vi "DL-Restore Configuration.vi"(11 "Error In":errorcluster) -> (8 "Config":T1={"Folder"=path "C:/Data", "Filestem"="Untitled", "Device"="", "Fs (Hz)"=50000.0, "T (s)"=120.0, "AI"=[], "frame size (s)"=1.0, ".wav file"=FALSE, "Trigger"=enum."Internal"}, 15 "error out":errorcluster)   [LabVIEW 2020]
uses:
  Typedefs/DL-Configuration.ctl
  Typedefs/DL-Channel Spec.ctl
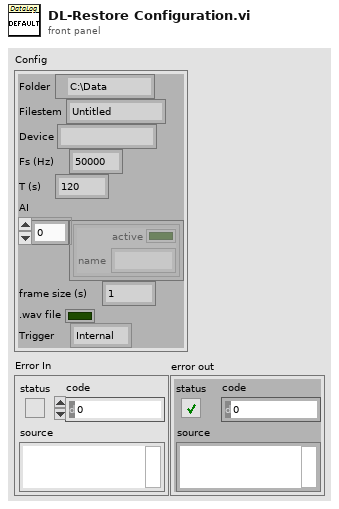
[diagram p1: front panel]
types:
  T1 = typedef "DL-Configuration.ctl" = cluster{"Folder":path, "Filestem":string, "Device":string, "Fs (Hz)":dbl, "T (s)":dbl, "AI":T2[], "frame size (s)":dbl, ".wav file":bool, "Trigger":enum16{"Internal", "External"}}
  T2 = typedef "DL-Channel Spec.ctl" = cluster{"active":bool, "name":string}
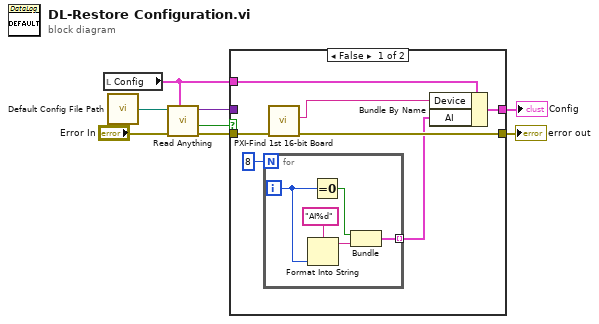
[diagram p0: block diagram]
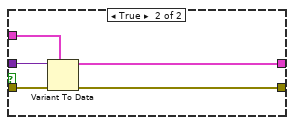
[diagram p2: hidden frame]
diagram:
  n1 = local read "Config"() -> (w3:T1)
  n2 = call "Default Config File Path.vi"() -> ("Default config file name"=w8:path)
  n3 = call "Read Anything.vi"("Type of Anything"=w3, "Error In"="Error In", "Path (dialog)"=w8) -> ("Error Out"=w4:errorcluster, "Found?"=w5:bool, "Anything"=w6:variant)  [unwired: 6 in]
  n4 = case shown="False" w5 {
    tunnel: w6 -> [_ w24]
    tunnel: w4 -> [w15 w25]
    tunnel: w3 -> [w14 w23]
    tunnel: [w12 w22] -> w2
    tunnel: [w11 w21] -> w1
    frame False {
      n5 = for {
        N: 8 -> [_]
        tunnel: [w16] -> w9 mode=indexing
        i -> [w18]
        n6 = Format Into String(format string="AI%d", w18) -> (resulting string=w19:string)  [unwired: 2 in, 1 out]
        n7 = Equal To 0?(x=w18) -> (x = 0?=w17:bool)
        n8 = Bundle(w17, w19) -> (w16:cluster{bool, string})  [unwired: 1 in]
      }
      n9 = call "PXI-Find 1st 16-bit Board.vi"("error in (no error)"=w15) -> ("error out"=w11:errorcluster, "DAQmx Device Name"=w13:tag)  [unwired: 8 in, 1 out]
      n10 = Bundle By Name(cluster=w14, "Device"=w13, "AI"=w9) -> (w12:T1)
    }
    frame True {
      n11 = Variant To Data(error in=w25, type=w23, Variant=w24) -> (data=w22:T1, error out=w21:errorcluster)
    }
  }
  "Config" <- w2
  "error out" <- w1
